vi "52-lfs-r4 begin.vi"(8 "error in (no error)":errorcluster, 9 "Position in":T1) -> (0 "error out":errorcluster, 1 "Position out":T1, 4 "side?":bool)   [LabVIEW 2019]
uses:
  subVI/move/position cluster.ctl
  subVI/move control/move and align/move_cluster.ctl
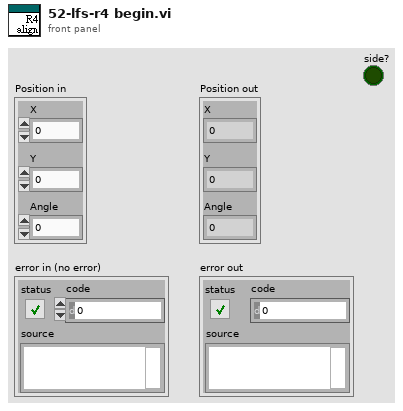
[diagram p1: front panel]
types:
  T1 = typedef "position cluster.ctl" = cluster{"X":dbl, "Y":dbl, "Angle":dbl}
  T2 = typedef "move_cluster.ctl" = cluster{"X":dbl, "Y":dbl, "degree":dbl, "speed":dbl}
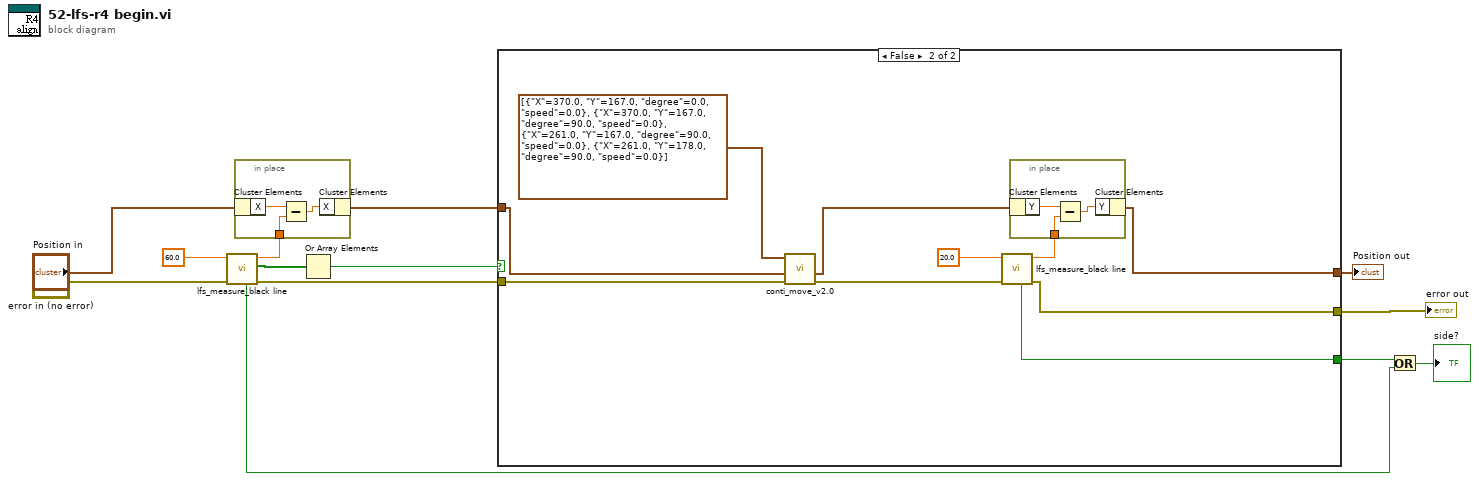
[diagram p0: block diagram]
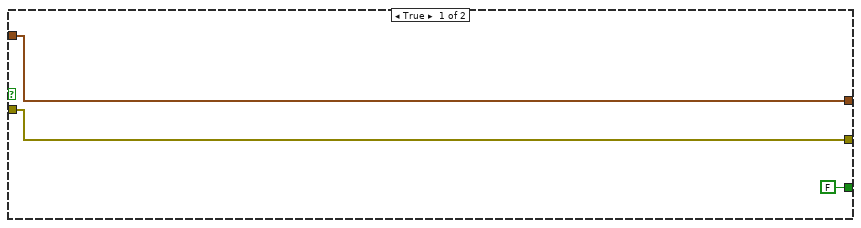
[diagram p2: hidden frame]
diagram:
  n1 = call "lfs_measure_black line.vi"("error in (no error)"="error in (no error)", "limit"=60.0) -> ("error out"=w6:errorcluster, "0:R 1:L"=w9:bool[], "move cm"=w10:dbl, "side?"=w2:bool)  [unwired: 6 in]
  n2 = in-place {
    in-place-border: w10 -> [w16]
    n3 = in-place-cluster #1("Position in") -> ("X"=w14:dbl)
    n4 = Subtract(x=w14, y=w16) -> (x-y=w15:dbl)
    n5 = in-place-cluster #1("X"=w15) -> (w7:T1)
  }
  n6 = Or Array Elements(Boolean array=w9) -> (logical OR=w8:bool)
  n7 = case shown="False" w8 {
    tunnel: w7 -> [w19 w28]
    tunnel: w6 -> [w18 w27]
    tunnel: [w18 w22] -> w5
    tunnel: [w19 w21] -> w4
    tunnel: [FALSE ("side?") w20] -> w3
    frame True {
    }
    frame False {
      n8 = call "conti_move_v2.0.vi"("error in (no error)"=w27, "Position"=w28, "route"=T2[] [{"X"=370.0, "Y"=167.0, "degree"=0.0, "speed"=0.0}, {"X"=370.0, "Y"=167.0, "degree"=90.0, "speed"=0.0}, {"X"=261.0, "Y"=167.0, "degree"=90.0, "speed"=0.0}, {"X"=261.0, "Y"=178.0, "degree"=90.0, "speed"=0.0}]) -> ("error out"=w23:errorcluster, "Position out"=w24:T1)  [unwired: 7 in]
      n9 = call "lfs_measure_black line.vi"("error in (no error)"=w23, "limit"=20.0) -> ("error out"=w22:errorcluster, "move cm"=w26:dbl, "side?"=w20:bool)  [unwired: 6 in, 1 out]
      n10 = in-place {
        in-place-border: w26 -> [w32]
        n11 = in-place-cluster #2(w24) -> ("Y"=w30:dbl)
        n12 = Subtract(x=w30, y=w32) -> (x-y=w31:dbl)
        n13 = in-place-cluster #2("Y"=w31) -> (w21:T1)
      }
    }
  }
  "error out" <- w5
  "Position out" <- w4
  n14 = Or(x=w3, y=w2) -> (x .or. y?=→"side?":bool)
